vi "Push Channel Analog.vi"(0 "ADALM2000 Handler":u32 caption="Instrument Handle Out", 1 "Channel":T1, 2 "data":dbl[](array[numeric])) -> (7 "ADALM2000 Handler 2":u32 caption="Instrument Handle Out")   [LabVIEW 2015]
uses:
  Controls/AnalogChannel.ctl
  libm2k_lv.dll
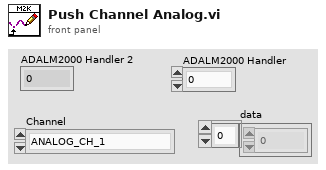
[diagram p1: front panel]
types:
  T1 = typedef "AnalogChannel.ctl" = enum16{"ANALOG_CH_1", "ANALOG_CH_2"}
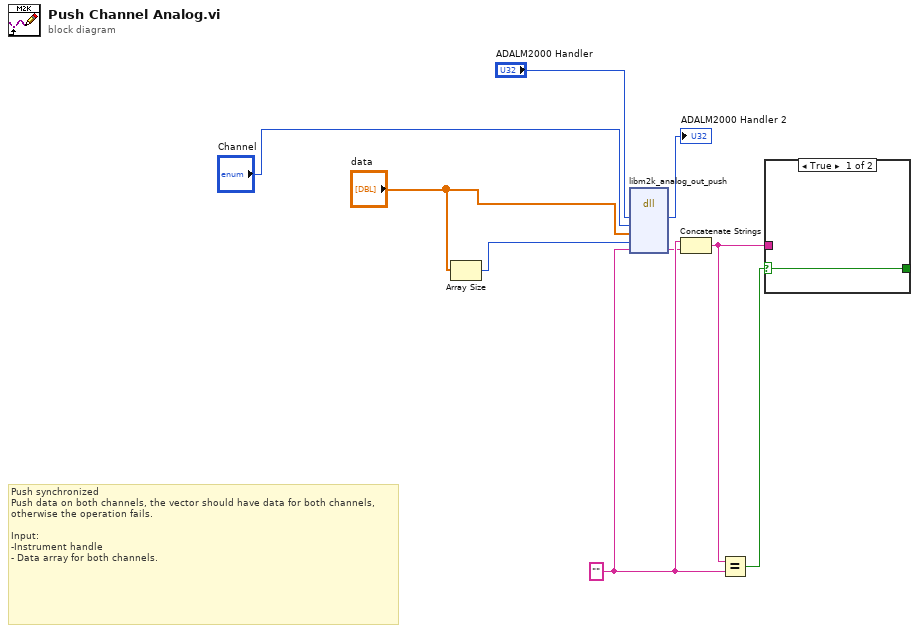
[diagram p0: block diagram]
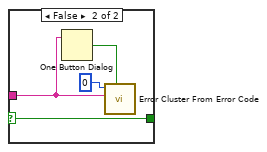
[diagram p2: hidden frame]
diagram:
  w9 = ""
  # "Push synchronized\nPush data on both channels, the vector should have data for both channels, otherwise the operation fails.\n\nInput:\n-Instrument handle\n- Data array for both channels."
  n1 = Array Size(array="data") -> (size(s)=w1:i32)
  n2 = dll-call lib="libm2k_lv.*" fn="libm2k_analog_out_push"("instance"="ADALM2000 Handler", "chnIdx"="Channel", "analog_samples"="data", "nb_samples"=w1, "err"=w9) -> ("instance"=→"ADALM2000 Handler 2":u64, "err"=w7:string)  [unwired: 7 in, 2 out]
  n3 = Concatenate Strings(w9, w7) -> (w5:string)
  n4 = Equal?(x=w5, y=w9) -> (x = y?=w6:bool)
  n5 = case shown="True" w6 {
    selector: w6 -> [w10 w11]
    tunnel: w5 -> [_ w13]
    tunnel: [w10 w11] -> _
    frame True {
    }
    frame False {
      n6 = One Button Dialog(message=w13) -> (true=w12:bool)  [unwired: 1 in]
      n7 = call <vilib>:"Error Cluster From Error Code.vi"("show call chain? (False)"=w12, "error message (\"\")"=w13, "error code (0)"=0) -> ()  [unwired: 6 in, 1 out]
    }
  }
